vi "DBLtoVariant.vi"(8 "error in":errorcluster, 10 "dataType":string, 11 "data":dbl) -> (0 "error out":errorcluster, 2 "variant out":variant, 3 "valid?":bool)   [LabVIEW 2020]
doc: "This VI converts <B>DBL</B> to the right type and then to <B>variant</B>. If none of the known data types or string is passed as variant, <B>valid</B> returns false."
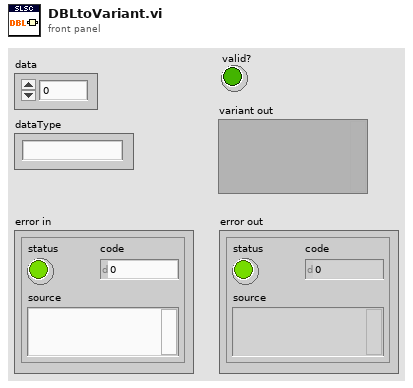
[diagram p1: front panel]
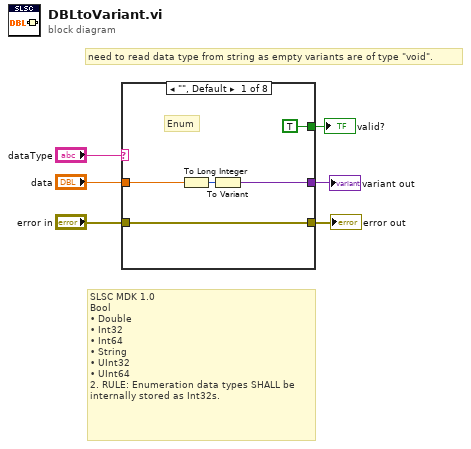
[diagram p0: block diagram]
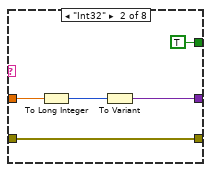
[diagram p2: hidden frame]
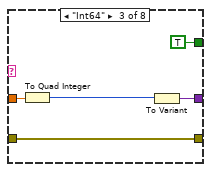
[diagram p3: hidden frame]
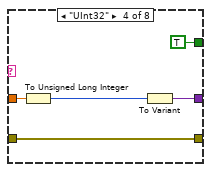
[diagram p4: hidden frame]
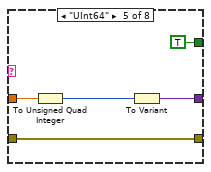
[diagram p5: hidden frame]
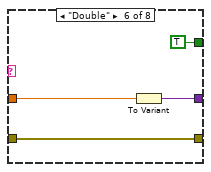
[diagram p6: hidden frame]
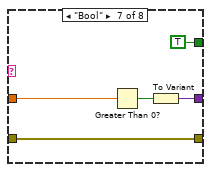
[diagram p7: hidden frame]
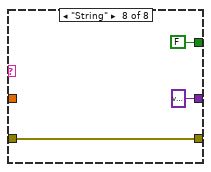
[diagram p8: hidden frame]
diagram:
  # "need to read data type from string as empty variants are of type \"void\"."
  # "SLSC MDK 1.0 \nBool\n• Double\n• Int32\n• Int64\n• String\n• UInt32\n• UInt64\n2. RULE: Enumeration data types SHALL be\ninternally stored as Int32s."
  n1 = case shown="\"\", Default" "dataType" {
    tunnel: "error in" -> [w11 w12 w21 w23 w27 w35 w40 w43]
    tunnel: [w11 w12 w21 w23 w27 w35 w40 w43] -> w6
    tunnel: [w7 w14 w18 w24 w28 w34 w36 variant ("Variant")] -> w2
    tunnel: "data" -> [w9 w16 w19 w26 w30 w33 w38 _]
    tunnel: [TRUE TRUE TRUE TRUE TRUE TRUE TRUE FALSE] -> w3
    frame "", Default {
      # "Enum"
      n2 = To Long Integer(number=w9) -> (32bit integer=w8:i32)
      n3 = To Variant(anything=w8) -> (Variant=w7:variant)
    }
    frame "Int32" {
      n4 = To Long Integer(number=w16) -> (32bit integer=w15:i32)
      n5 = To Variant(anything=w15) -> (Variant=w14:variant)
    }
    frame "Int64" {
      n6 = To Quad Integer(1:w19) -> (0:w17:i64)
      n7 = To Variant(anything=w17) -> (Variant=w18:variant)
    }
    frame "UInt32" {
      n8 = To Unsigned Long Integer(number=w26) -> (unsigned 32bit integer=w25:u32)
      n9 = To Variant(anything=w25) -> (Variant=w24:variant)
    }
    frame "UInt64" {
      n10 = To Unsigned Quad Integer(1:w30) -> (0:w29:u64)
      n11 = To Variant(anything=w29) -> (Variant=w28:variant)
    }
    frame "Double" {
      n12 = To Variant(anything=w33) -> (Variant=w34:variant)
    }
    frame "Bool" {
      n13 = Greater Than 0?(x=w38) -> (x > 0?=w37:bool)
      n14 = To Variant(anything=w37) -> (Variant=w36:variant)
    }
    frame "String" {
    }
  }
  "error out" <- w6
  "variant out" <- w2
  "valid?" <- w3
